vi "ziGetValueDemodSample.vi"(4 "error in":errorcluster, 5 "Demod Sample In":T1, 6 "Path":string, 7 "Handle In":T2 {"Handle" format="0x%08x"; "Conn" format="0x%08x"}) -> (0 "error out":errorcluster, 1 "Demod Sample Out":T1, 3 "Handle Out":T2 {"Handle" format="0x%08x"; "Conn" format="0x%08x"})   [LabVIEW 2016, in "Zurich Instruments LabOne.lvlib"]
doc: "This function retrieves the newest available sample from a demodulator's sample node. The value first found is returned if more than one value is available (a wildcard is used in the path). This function is only applicable to paths matching DEMODS/[0-9]+/SAMPLE."
uses:
  Zurich Instruments LabOne.lvlib
  ziTypeHandle.ctl
  Zurich Instruments/LabOne/API/LabVIEW/Zurich Instruments LabOne/Private/ziLV64.framework
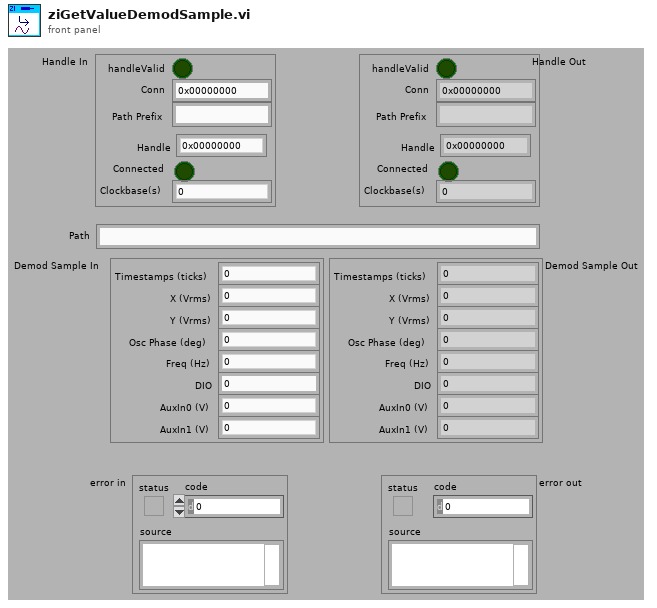
[diagram p1: front panel]
types:
  T1 = cluster{"Timestamps (ticks)":u64, "X (Vrms)":dbl, "Y (Vrms)":dbl, "Osc Phase (deg)":dbl, "Freq (Hz)":dbl, "DIO":u32, "AuxIn0 (V)":dbl, "AuxIn1 (V)":dbl}
  T2 = typedef "Zurich Instruments LabOne.lvlib/ziTypeHandle.ctl" = cluster{"handleValid":bool, "Conn":u64, "Path Prefix":string, "Handle":u64, "Connected":bool, "Clockbase(s)":dbl}
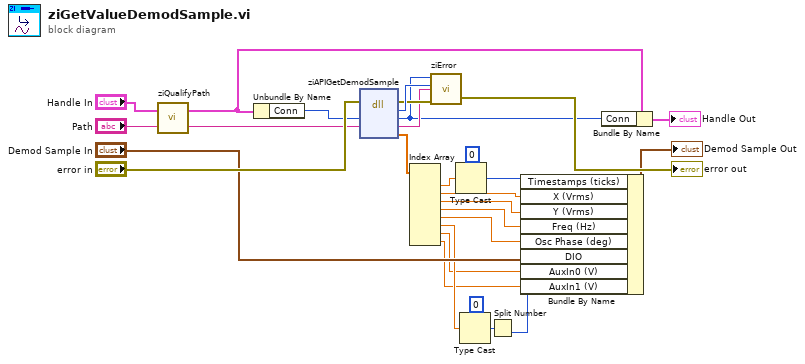
[diagram p0: block diagram]
diagram:
  n1 = call "ziQualifyPath.vi"("Path In"="Path", "Handle In"="Handle In") -> ("Path Out"=w21:string, "Handle Out"=w19:T2)
  n2 = Unbundle By Name(w19) -> ("Conn"=w27:u64)
  n3 = dll-call lib="Users/arkady/Desktop/ado/github/resonant_ultrasound_arxiv/maglab ultrasound -- arkady --arxiv/Zurich Instruments/LabOne/API/LabVIEW/Zurich Instruments LabOne/Private/ziLV*.*" fn="ziAPIGetDemodSample" label="ziAPIGetValueS"(error in="error in", "Conn"=w27, "Path"=w21) -> (error out=w25:errorcluster, "return type"=w26:u32, "Conn"=w1:u64, "Path"=w18:string, "DemodSample"=w11:dbl[])  [unwired: 2 in, 2 out]
  n4 = Index Array(array=w11) -> (element #1=w3:dbl, element #2=w13:dbl, element #3=w14:dbl, element #4=w15:dbl, element #5=w16:dbl, element #6=w9:dbl, element #7=w8:dbl, element #8=w7:dbl)  [unwired: 8 in]
  n5 = call "ziError.vi"("Conn"=w1, "ziErrorCode"=w26, "Error In"=w25, "Annotation"=w18) -> ("Error Out"=→"error out":errorcluster)  [unwired: 1 in, 1 out]
  n6 = Type Cast(type=u64 0 ("DIO"), x=w3) -> (*(type *) &x=w2:u64)
  n7 = Type Cast(type=u64 0 ("DIO"), x=w9) -> (*(type *) &x=w6:u64)
  n8 = Split Number(x=w6) -> (lo(x)=w5:u32)  [unwired: 1 out]
  n9 = Bundle By Name(cluster="Demod Sample In", "Timestamps (ticks)"=w2, "X (Vrms)"=w13, "Y (Vrms)"=w14, "Freq (Hz)"=w15, "Osc Phase (deg)"=w16, "DIO"=w5, "AuxIn0 (V)"=w8, "AuxIn1 (V)"=w7) -> (→"Demod Sample Out":T1)
  n10 = Bundle By Name(cluster=w19, "Conn"=w1) -> (→"Handle Out":T2)
